vi "Read Max Power.vi"(8 "错误输入（无错误）":errorcluster, 10 "Delay":u32=8000, 11 "OSC Input":refnum<visa-resource-name>) -> (0 "错误输出":errorcluster, 2 "Pace Max Amp":dbl, 3 "OSC Output":refnum<visa-resource-name>)   [LabVIEW 2016]
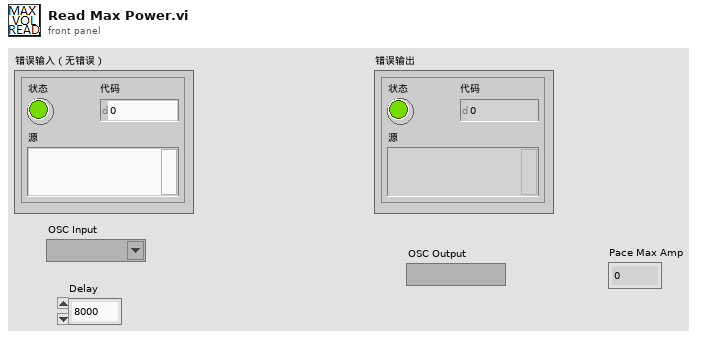
[diagram p1: front panel]
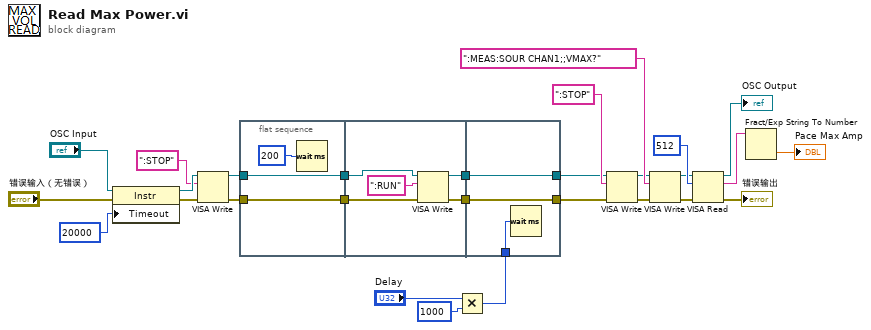
[diagram p0: block diagram]
diagram:
  n1 = property class="Instr"(reference="OSC Input", error in="错误输入（无错误）", "Timeout"=u32 20000 ("General Settings:Timeout Value")) -> (reference out=w17:refnum<visa-resource-name>, error out=w15:errorcluster)
  n2 = VISA Write(VISA resource name=w17, write buffer=":STOP" ("写入缓冲区"), error in (no error)=w15) -> (VISA resource name out=w7:refnum<visa-resource-name>, error out=w6:errorcluster)  [unwired: 1 out]
  n3 = flat-sequence {
    tunnel: w6 -> [w30]
    tunnel: w7 -> [w31]
    tunnel: [w31] -> w2
    tunnel: [w30] -> w1
    tunnel: [w35] -> w5
    tunnel: [w34] -> w4
    tunnel: w2 -> [w33]
    tunnel: w1 -> [w32]
    tunnel: [w38] -> w8
    tunnel: [w39] -> w9
    tunnel: w5 -> [w39]
    tunnel: w4 -> [w38]
    tunnel: w3 -> [w37]
    frame #0 {
      n4 = Wait (ms)(milliseconds to wait=u32 200 ("等待时间（毫秒）")) -> ()  [unwired: 1 out]
    }
    frame #1 {
      n5 = VISA Write(VISA resource name=w33, write buffer=":RUN" ("写入缓冲区"), error in (no error)=w32) -> (VISA resource name out=w35:refnum<visa-resource-name>, error out=w34:errorcluster)  [unwired: 1 out]
    }
    frame #2 {
      n6 = Wait (ms)(milliseconds to wait=w37) -> ()  [unwired: 1 out]
    }
  }
  n7 = Multiply(x="Delay", y=u32 1000) -> (x*y=w3:u32)
  n8 = VISA Write(VISA resource name=w9, write buffer=":STOP" ("写入缓冲区"), error in (no error)=w8) -> (VISA resource name out=w11:refnum<visa-resource-name>, error out=w10:errorcluster)  [unwired: 1 out]
  n9 = VISA Write(VISA resource name=w11, write buffer=":MEAS:SOUR CHAN1;;VMAX?" ("写入缓冲区"), error in (no error)=w10) -> (VISA resource name out=w25:refnum<visa-resource-name>, error out=w24:errorcluster)  [unwired: 1 out]
  n10 = VISA Read(VISA resource name=w25, byte count=u32 512 ("字节总数"), error in (no error)=w24) -> (VISA resource name out=→"OSC Output":refnum<visa-resource-name>, read buffer=w23:string, error out=→"错误输出":errorcluster)  [unwired: 1 out]
  n11 = Fract/Exp String To Number(string=w23) -> (number=→"Pace Max Amp":dbl)  [unwired: 3 in, 1 out]
